vi "Write.vi"(8 "error in (no error)":errorcluster, 10 "command":string, 11 "HAL.Serial in":refnum<class "HAL.Serial.lvclass">) -> (0 "error out":errorcluster, 3 "HAL.Serial out":refnum<class "HAL.Serial.lvclass">)   [LabVIEW 2019, in "HAL.Serial.lvclass"]
doc: "Override to <b>open</b> a connection to your instrument."
uses:
  HAL.Serial.lvclass
  HAL.Serial.lvclass/HAL.Serial.ctl
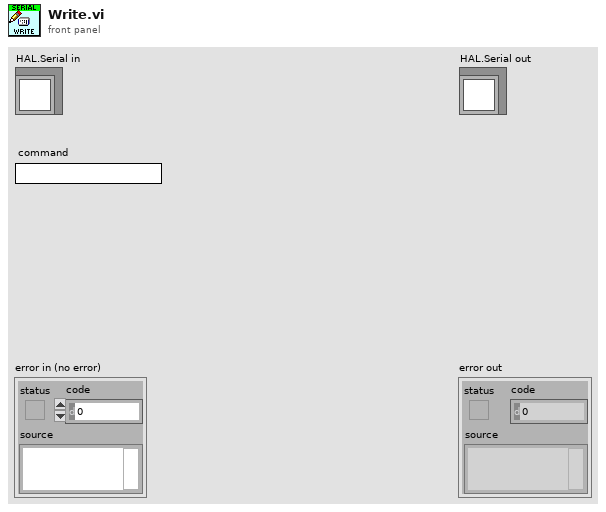
[diagram p1: front panel]
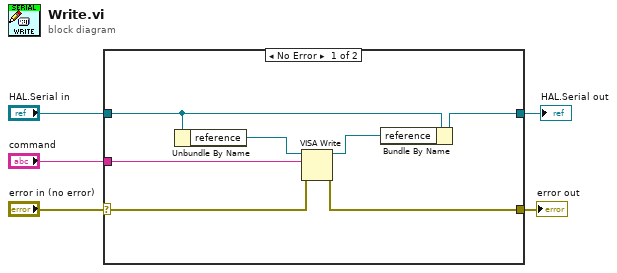
[diagram p0: block diagram]
diagram:
  n1 = case shown="No Error" "error in (no error)" {
    selector: "error in (no error)" -> [w12 w14]
    tunnel: [w11 w14] -> w5
    tunnel: "HAL.Serial in" -> [w8 w13]
    tunnel: "command" -> [w9 _]
    tunnel: [w7 w13] -> w1
    frame No Error {
      n2 = Unbundle By Name(w8) -> ("reference"=w10:refnum<visa-resource-name>)
      n3 = VISA Write(VISA resource name=w10, write buffer=w9, error in (no error)=w12) -> (VISA resource name out=w6:refnum<visa-resource-name>, error out=w11:errorcluster)  [unwired: 1 out]
      n4 = Bundle By Name(cluster=w8, "reference"=w6) -> (w7:refnum<class "HAL.Serial.lvclass">)
    }
    frame Error {
    }
  }
  "error out" <- w5
  "HAL.Serial out" <- w1
